vi "Safe Date-Time String.vi"(2 "local BR/TU (BR)":bool, 4 "ano 4ou2 digitos (4)":bool) -> (0 "Safe time string":string, 1 "Safe date string":string, 3 "Precise time string":string)   [LabVIEW 2018]
panel:
  # "TERMINAL DE SAÍDA Precise time string CONECTADO \nTEMPORARIAMENTE NO LADO ESQUERDO DO VI PARA \nFAZER TESTES SEM QUEBRAR TODAS AS INSTÂNCIAS DESTE VI."
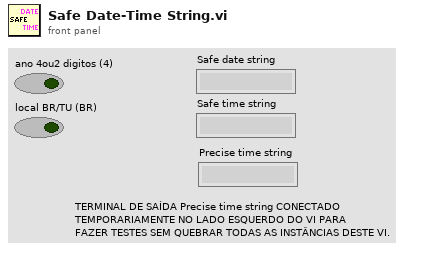
[diagram p1: front panel]
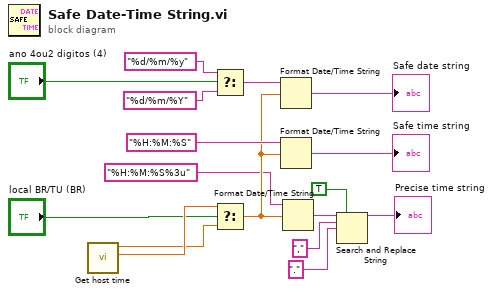
[diagram p0: block diagram]
diagram:
  n1 = call "Get host time.vi"() -> ("TU time"=w12:dbl, "BR time"=w11:dbl)  [unwired: 8 in, 2 out]
  n2 = Select(t="%d/%m/%y" ("time format string (%c)"), s="ano 4ou2 digitos (4)", f="%d/%m/%Y" ("time format string (%c)")) -> (s? t:f=w13:string)
  n3 = Select(t=w12, s="local BR/TU (BR)", f=w11) -> (s? t:f=w7:dbl)
  n4 = Format Date/Time String(time format string (%c)=w13, seconds (now)=w7) -> (date/time string=→"Safe date string":string)  [unwired: 1 in]
  n5 = Format Date/Time String(time format string (%c)="%H:%M:%S", seconds (now)=w7) -> (date/time string=→"Safe time string":string)  [unwired: 1 in]
  n6 = Format Date/Time String(time format string (%c)="%H:%M:%S%3u", seconds (now)=w7) -> (date/time string=w5:string)  [unwired: 1 in]
  n7 = Search and Replace String(replace all?=TRUE ("replace all? (F)"), input string=w5, search string=",", replace string="." ("replace string (\"\")")) -> (result string=→"Precise time string":string)  [unwired: 4 in, 3 out]
